vi "LVClass_WavefrontCorrectorSet Get WavefrontCorrectorSpecification.vi"(0 "WavefrontCorrectorSet in":refnum<class "WavefrontCorrectorSet.lvclass">, 11 "error in (no error)":errorcluster) -> (4 "WavefrontCorrectorSet out":refnum<class "WavefrontCorrectorSet.lvclass">, 6 "ConfigMiroir":T1={"Mirror name"="", "Plugin name"="", "Serial number"="", "Revision"="", "Number of commands"=0, "Sleep after command apply (ms)"=0, "Has internal memory ?"=TRUE}, 15 "error out":errorcluster)   [LabVIEW 2020, in "WavefrontCorrectorSet.lvclass"]
doc: "WavefrontCorrector specifications getters.\n\n--------------------------------------------------------------------------------\n\n<B>wavefrontcorrector_setIn </B> : WavefrontCorrectorSet object.\n<B>wavefrontcorrector_setOut </B> : WavefrontCorrectorSet object.\n<B>driver_name </B> : Wavefront corrector driver name.\n<B>wavefrontcorrector_name </B> : Wavefront corrector pretty name.\n<B>wavefrontcorrector_serial_number</B> : Wavefront corrector serial number.\n<B>revision </B> : Wavefront corrector revision.\n<B>actuators_count </B> : Wavefront corrector actuators count.\n<B>min_sleep_after_movement </B> : Wavefront corrector actuators stabilization delay.\n<B>ErrorIn </B> : Error\n<B>ErrorOut </B> : Error\n\n--------------------------------------------------------------------------------"
uses:
  WavefrontCorrectorSet.lvclass
  WavefrontCorrectorSpecifications.ctl
  WavefrontCorrectorSet.lvclass/WavefrontCorrectorSet.ctl
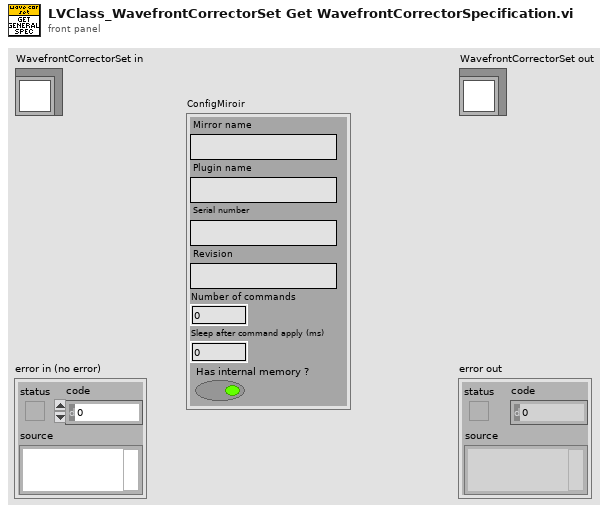
[diagram p1: front panel]
types:
  T1 = typedef "WavefrontCorrectorSpecifications.ctl" = cluster{"Mirror name":string, "Plugin name":string, "Serial number":string, "Revision":string, "Number of commands":i32, "Sleep after command apply (ms)":i32, "Has internal memory ?":bool}
  T2 = typedef "ClassID.ctl" = i64
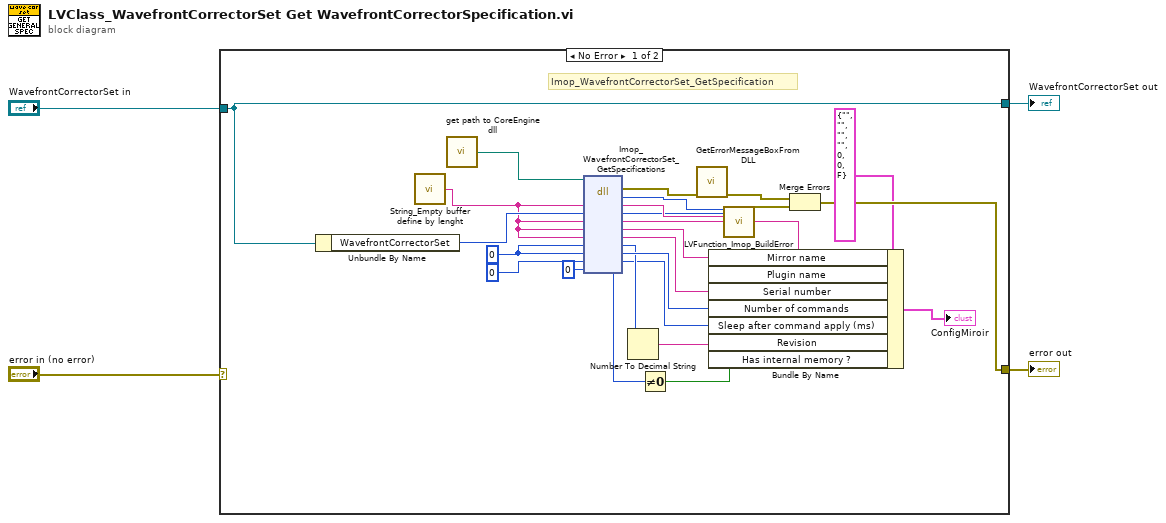
[diagram p0: block diagram]
diagram:
  n1 = case shown="No Error" "error in (no error)" {
    selector: "error in (no error)" -> [_ w31]
    tunnel: [w27 w31] -> w1
    tunnel: [w26 w30] -> w2
    tunnel: "WavefrontCorrectorSet in" -> [w26 w30]
    frame No Error {
      w12 = 0 ("nb_actuator")
      # "Imop_WavefrontCorrectorSet_GetSpecification"
      n2 = Unbundle By Name(w26) -> ("WavefrontCorrectorSet"=w24:T2)
      n3 = call "String_Empty buffer define by lenght.vi"() -> ("Empty buffer"=w20:string)  [unwired: 1 in]
      n4 = call "get path to CoreEngine dll.vi"() -> ("path to wavekit library"=w25:path)  [unwired: 14 in, 1 out]
      n5 = dll-call lib="D:/soft/HASO_v3/SVN_trunk/ImOpCoreEngine4_LV2011/DLLs/c_interface_vc100.dll" fn="Imop_WavefrontCorrectorSet_GetSpecifications"(path in=w25, "message"=w20, "WavefrontCorrectionSet"=w24, "driver_name"=w20, "WaveFrontCorrector_name"=w20, "WaveFrontCorrector_serial_number"=w20, "revision"=w12, "nb_actuator"=w12, "min_sleep_after_movement"=0, "Has internal memory"=u8 0) -> (error out=w23:errorcluster, "return type"=w22:i32, "message"=w21:string, "WavefrontCorrectionSet"=w5:i64, "driver_name"=w13:string, "WaveFrontCorrector_name"=w17:string, "WaveFrontCorrector_serial_number"=w15:string, "revision"=w11:i32, "nb_actuator"=w14:i32, "min_sleep_after_movement"=w9:i32, "Has internal memory"=w8:u8)  [unwired: 2 in, 1 out]
      n6 = Number To Decimal String(number=w11) -> (decimal integer string=w10:string)  [unwired: 1 in]
      n7 = Not Equal To 0?(x=w8) -> (x != 0?=w7:bool)
      n8 = call "GetErrorMessageBoxFromDLL.vi"("error IN"=w23) -> ("error OUT"=w29:errorcluster)  [unwired: 10 in]
      n9 = Bundle By Name(cluster=T1 {"Mirror name"="", "Plugin name"="", "Serial number"="", "Revision"="", "Number of commands"=0, "Sleep after command apply (ms)"=0, "Has internal memory ?"=FALSE} ("ConfigMiroir"), "Mirror name"=w17, "Plugin name"=w13, "Serial number"=w15, "Number of commands"=w14, "Sleep after command apply (ms)"=w9, "Revision"=w10, "Has internal memory ?"=w7) -> (→"ConfigMiroir":T1)
      n10 = call "LVFunction_Imop_BuildError.vi"("code"=w22, "String to Prepend to source (\"\")"=w21, "Adresse"=w5) -> ("error out"=w28:errorcluster)  [unwired: 12 in]
      n11 = Merge Errors(w29, w28) -> (w27:errorcluster)
    }
    frame Error {
    }
  }
  "error out" <- w1
  "WavefrontCorrectorSet out" <- w2
